vi "Append Horizontal Line to Report.vi"(0 "report in":refnum<class "NI_HTML.lvclass">, 1 "size (default)":i32=1, 2 "MS Office parameters":T2, 5 "align (default)":T1, 9 "width (100=default)":dbl=100.0 format="%.2f", 11 "error in (no error)":errorcluster, 12 "width units (Percentage)":enum16{"Pixels", "Percentage"}(ring)=enum."Percentage", 13 "noshade (F)":bool) -> (4 "report out":refnum<class "NI_HTML.lvclass">, 15 "error out":errorcluster)   [LabVIEW 2015, in "NI_HTML.lvclass"]
doc: "Creates a horizontal rule in an HTML, Word, or Excel report. You cannot use this VI with standard reports."
uses:
  <vilib>/Utility/NIReport.llb/HTML/NI_HTML.lvclass
  <vilib>/Utility/NIReport.llb/HTML Report Text Alignment.ctl
  <vilib>/Utility/NIReport.llb/HTML/NI_HTML.lvclass/NI_HTML.ctl
  <vilib>/Utility/NIReport.llb/NI_ReportGenerationCore.lvlib
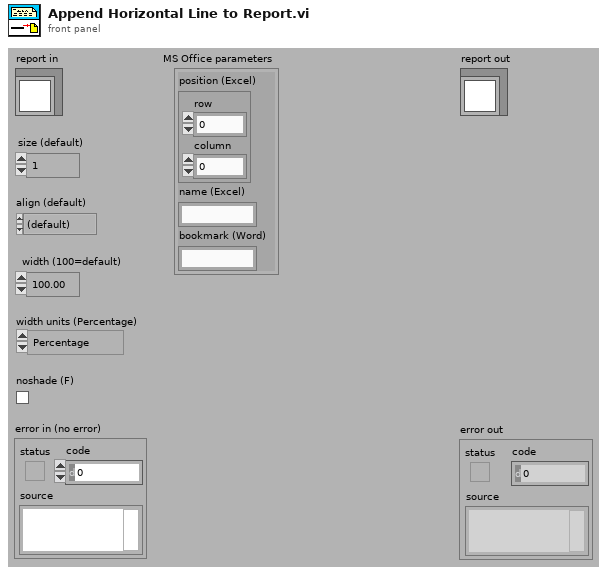
[diagram p1: front panel]
types:
  T1 = typedef "NI_ReportGenerationCore.lvlib/HTML Report Text Alignment.ctl" = enum16{"(default)", "LEFT", "CENTER", "RIGHT"}
  T2 = cluster{"position (Excel)":cluster{"row":i32, "column":i32}, "name (Excel)":string, "bookmark (Word)":string}
  T3 = typedef "NI_ReportGenerationCore.lvlib/HTML Report Data.ctl" = cluster{"Body Text":string, "Font Tag":string, "Title Text":string, "Header Text":string, "Footer Text":string, "Image List":path[]}
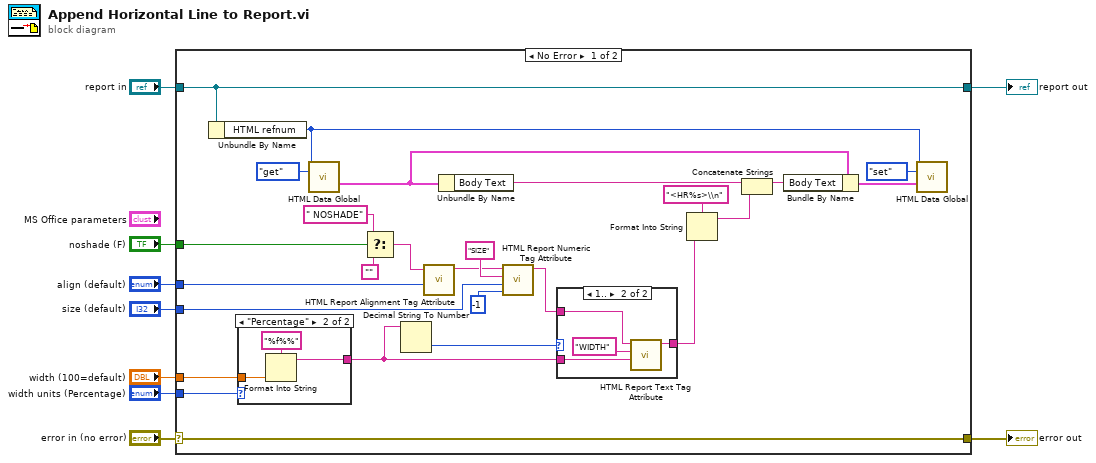
[diagram p0: block diagram]
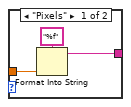
[diagram p3: hidden frame]
diagram:
  n1 = case shown="No Error" "error in (no error)" {
    selector: "error in (no error)" -> [w35 w48]
    tunnel: [w35 w48] -> w8
    tunnel: [w14 w47] -> w6
    tunnel: "report in" -> [w14 w47]
    tunnel: "width units (Percentage)" -> [w20 _]
    tunnel: "width (100=default)" -> [w19 _]
    tunnel: "size (default)" -> [w18 _]
    tunnel: "align (default)" -> [w17 _]
    tunnel: "noshade (F)" -> [w16 _]
    frame No Error {
      n2 = Unbundle By Name(w14) -> ("HTML refnum"=w10:u32)
      n3 = case shown="\"Percentage\"" w20 {
        tunnel: w19 -> [w43 w46]
        tunnel: [w42 w45] -> w23
        frame "Pixels" {
          n4 = Format Into String(format string="%f" ("Format String"), w43) -> (resulting string=w42:string)  [unwired: 2 in, 1 out]
        }
        frame "Percentage" {
          n5 = Format Into String(format string="%f%%" ("Format String"), w46) -> (resulting string=w45:string)  [unwired: 2 in, 1 out]
        }
      }
      n6 = call <vilib>:"HTML Data Global.vi"("HTML refnum"=w10, "menu"=enum16{"init", "get", "set", "delete"}."get") -> ("HTML report data out"=w11:T3)  [unwired: 1 in, 12 out]
      n7 = Select(t=" NOSHADE", s=w16, f="") -> (s? t:f=w31:string)
      n8 = Decimal String To Number(string=w23) -> (number=w34:i32)  [unwired: 3 out]
      n9 = call <vilib>:"HTML Report Alignment Tag Attribute.vi"("align (default)"=w17, "tag attributes in"=w31) -> ("tag attributes out"=w25:string)  [unwired: 5 out]
      n10 = Unbundle By Name(w11) -> ("Body Text"=w21:string)
      n11 = call <vilib>:"HTML Report Numeric Tag Attribute.vi"("default value (0)"=-1, "value"=w18, "label"="SIZE", "tag attributes in"=w25) -> ("tag attributes out"=w28:string)  [unwired: 3 out]
      n12 = case shown="1.." w34 {
        tunnel: w28 -> [w36 w40]
        tunnel: [w36 w38] -> w29
        tunnel: w23 -> [_ w37]
        frame ..0 {
        }
        frame 1.. {
          n13 = call <vilib>:"HTML Report Text Tag Attribute.vi"("value"=w37, "label"="WIDTH", "tag attributes in"=w40) -> ("tag attributes out"=w38:string)  [unwired: 1 in, 3 out]
        }
      }
      n14 = Format Into String(format string="<HR%s>\\n", w29) -> (resulting string=w32:string)  [unwired: 2 in, 1 out]
      n15 = Concatenate Strings(w21, w32) -> (w22:string)
      n16 = Bundle By Name(cluster=w11, "Body Text"=w22) -> (w12:T3)
      n17 = call <vilib>:"HTML Data Global.vi"("HTML refnum"=w10, "menu"=enum16{"init", "get", "set", "delete"}."set", "HTML report data in"=w12) -> ()  [unwired: 13 out]
    }
    frame Error {
    }
  }
  "error out" <- w8
  "report out" <- w6
